vi "Handle Incoming Packets.vi"(8 "error in (no error)":errorcluster, 9 "SessionMailbox":refnum<queue>, 10 "Incoming Packet":refnum<class "ControlPacket.lvclass">, 11 "MQTT_Base in":refnum<class "MQTT_Base.lvclass">) -> (0 "error out":errorcluster, 1 "SessionMailbox out":refnum<queue>, 2 "Outgoing":T1, 3 "MQTT_Base out":refnum<class "MQTT_Base.lvclass">)   [LabVIEW 2013, in "MQTT Base.lvlib" / "MQTT_Base.lvclass"]
uses:
  MQTT_Base.lvclass
  <vilib>/LabVIEW Open Source Project/MQTT Control Packets/Control Packets/ControlPacket/ControlPacket.lvclass
  Response -- cluster.ctl
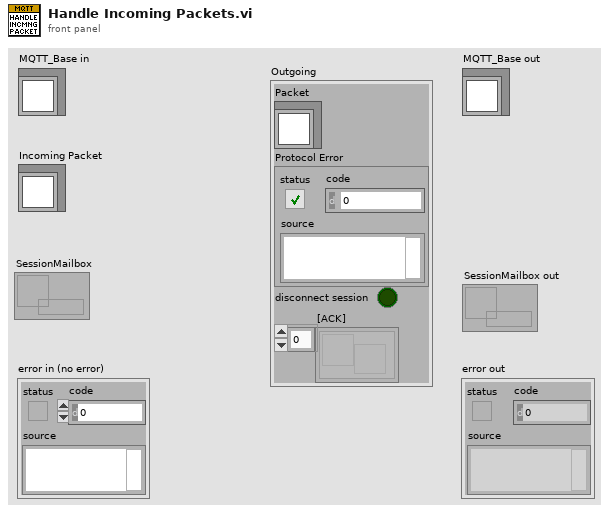
[diagram p1: front panel]
types:
  T1 = typedef "MQTT Base.lvlib/MQTT_Base.lvclass/Response -- cluster.ctl" = cluster{"Packet":refnum<class "ControlPacket.lvclass">, "Protocol Error":errorcluster, "disconnect session":bool, "[ACK]":refnum<notifier>[]}
  T2 = typedef "MQTT_Control_Packets.lvlib/ControlPacket.lvclass/Control Packet Type -- enum.ctl" = enum16{"Reserved", "CONNECT", "CONNACK", "PUBLISH", "PUBACK", "PUBREC", "PUBREL", "PUBCOMP", "SUBSCRIBE", "SUBACK", "UNSUBSCRIBE", "UNSUBACK", "PINGREQ", "PINGRESP", "DISCONNECT", "AUTH"}
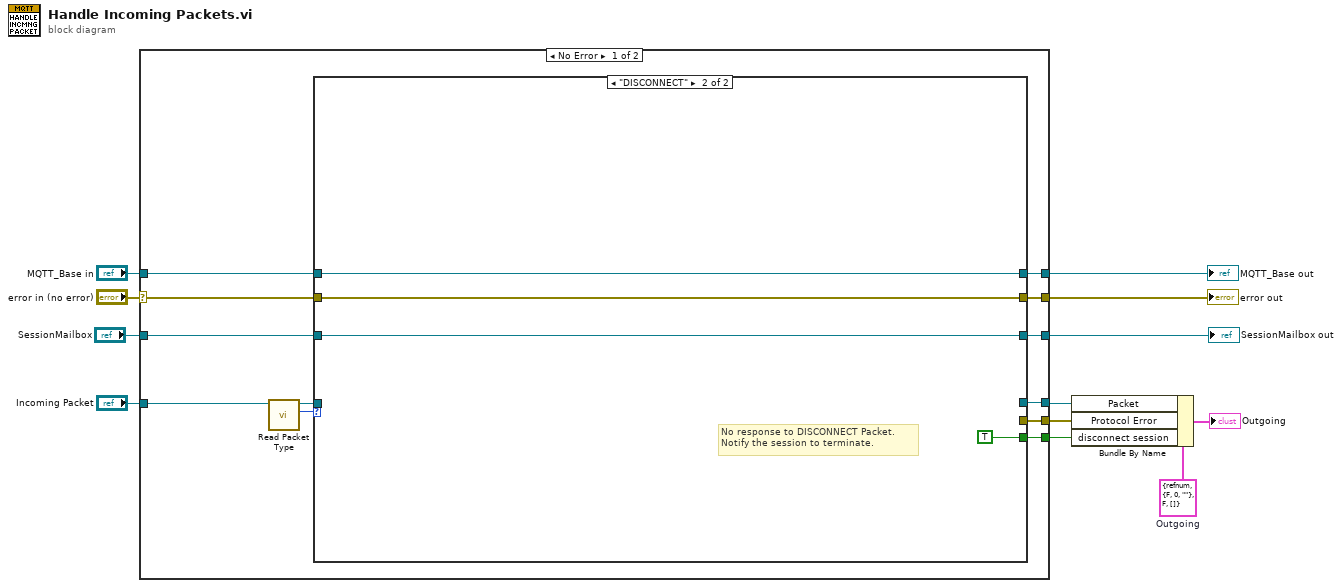
[diagram p0: block diagram]
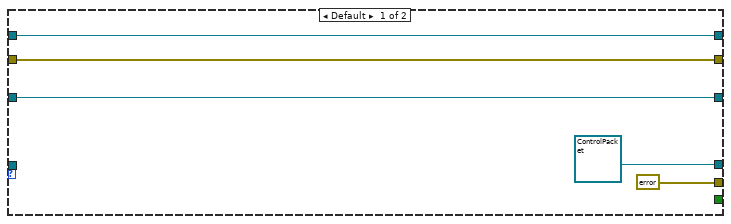
[diagram p2: hidden frame]
diagram:
  w7 = T1 {"Packet"=refnum, "Protocol Error"={"status"=FALSE, "code"=0, "source"=""}, "disconnect session"=FALSE, "[ACK]"=[]}  # Outgoing
  n1 = case shown="No Error" "error in (no error)" {
    selector: "error in (no error)" -> [w22 w36]
    tunnel: [w19 w36] -> w11
    tunnel: [w20 w35] -> w9
    tunnel: "MQTT_Base in" -> [w21 w35]
    tunnel: "Incoming Packet" -> [w15 _]
    tunnel: [w18 _] -> w6
    tunnel: [w17 _] -> w2
    tunnel: "SessionMailbox" -> [w16 w34]
    tunnel: [w14 w34] -> w1
    tunnel: [w13 _] -> w4
    frame No Error {
      n2 = call <vilib>:"Read Packet Type.vi"("ControlPacket in"=w15) -> ("Control Packet Type"=w24:T2, "ControlPacket out"=w23:refnum<class "ControlPacket.lvclass">)  [unwired: 9 in]
      n3 = case shown="\"DISCONNECT\"" w24 {
        tunnel: w23 -> [_ _]
        tunnel: w22 -> [w28 w32]
        tunnel: w21 -> [w29 w33]
        tunnel: [w29 w33] -> w20
        tunnel: [w28 w32] -> w19
        tunnel: w16 -> [w26 w30]
        tunnel: [refnum<class "ControlPacket.lvclass"> refnum ("ServerResponse") _] -> w18
        tunnel: [errorcluster {"status"=FALSE, "code"=0, "source"=""} ("error IO") _] -> w17
        tunnel: [w26 w30] -> w14
        tunnel: [_ TRUE ("disconnect")] -> w13
        frame Default {
        }
        frame "DISCONNECT" {
          # "No response to DISCONNECT Packet.\nNotify the session to terminate."
        }
      }
    }
    frame Error {
    }
  }
  "error out" <- w11
  "MQTT_Base out" <- w9
  "SessionMailbox out" <- w1
  n4 = Bundle By Name(cluster=w7, "Packet"=w6, "Protocol Error"=w2, "disconnect session"=w4) -> (→"Outgoing":T1)
